vi "RxCalOff.vi"(8 "error in (no error)":errorcluster, 11 "VISA":string) -> (0 "error out":errorcluster)   [LabVIEW 2015]
uses:
  RXCalDLL.dll
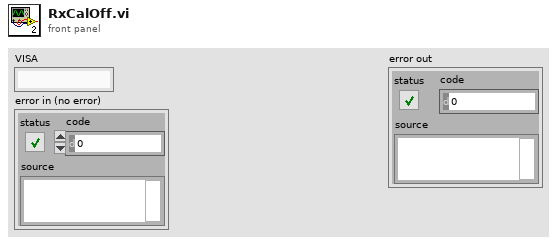
[diagram p1: front panel]
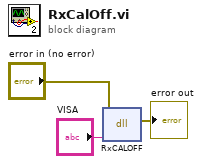
[diagram p0: block diagram]
diagram:
  n1 = dll-call lib="D:/4-Up-WLAN-Test-System/WTSInstrumentControl/rx cal/RXCalDLL.dll" fn="RxCALOFF"(error in="error in (no error)", "VISA"="VISA") -> (error out=→"error out":errorcluster)  [unwired: 4 in, 1 out]
